vi "Create and Map Output Channel.vi"(8 "error in (no error)":errorcluster, 9 "Tag Name":string, 10 "engine":refnum<data-value>, 11 "E2E editor node in":refnum<data-value>) -> (0 "error out":errorcluster, 2 "engine out":refnum<data-value>, 3 "E2E editor node out":refnum<data-value>)   [LabVIEW 2015, in "E2E Tag Exchange editor node.lvclass"]
uses:
  E2E Tag Exchange editor node.lvclass
  <vilib>/NI/DCAF/Tag Editor Core/Configuration Editor/Classes/Engine Parent/Engine Parent Editor Node.lvclass
  <vilib>/NI/Tag Bus Module Framework/channel/channel classification.ctl
  E2E Tag Exchange editor node.lvclass/E2E Tag Exchange editor node.ctl
  <vilib>/NI/Tag Bus/tag/tag descriptor.lvclass/tag descriptor.ctl
  <vilib>/NI/Configuration Framework/serializable configuration/NISE_CEF_serializable configuration.lvclass/NISE_CEF_serializable configuration.ctl
  <vilib>/Utility/LVClass/Get LV Class Name.vi
  <vilib>/NI/Configuration Framework/error generator/NISE_error generator.vi
  <vilib>/NI/Module Execution Interface/Engine Configuration/engine configuration.lvclass
  module/configuration/E2E Tag Exchange configuration.lvclass
  <vilib>/NI/Tag Bus Module Framework/channel/TBM channel.lvclass
  <vilib>/NI/Tag Bus/tag/tag descriptor.lvclass
  <vilib>/NI/Configuration Framework/serializable configuration/NISE_CEF_serializable configuration.lvclass
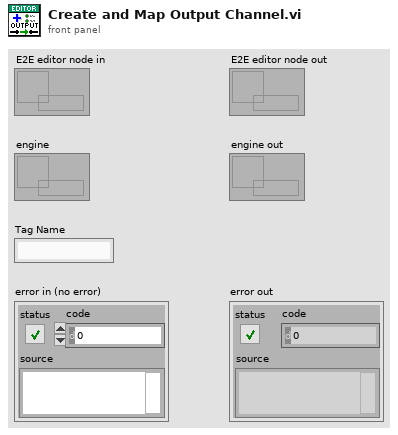
[diagram p1: front panel]
types:
  T1 = typedef "TBM channel.lvclass/channel classification.ctl" = enum16{"input data", "output data", "processing parameter", "processing result"}
  T2 = typedef "tag bus.lvlib/tag descriptor.lvclass/Data Type.ctl" = enum16{"Double", "Single", "I64", "I32", "I16", "I8", "U64", "U32", "U16", "U8", "Boolean", "String", "Array of Double", "Array of Single", "Array of I64", "Array of I32", "Array of I16", "Array of I8", "Array of U64", "Array of U32", "Array of U16", "Array of U8", "Array of Boolean", "Array of String"}
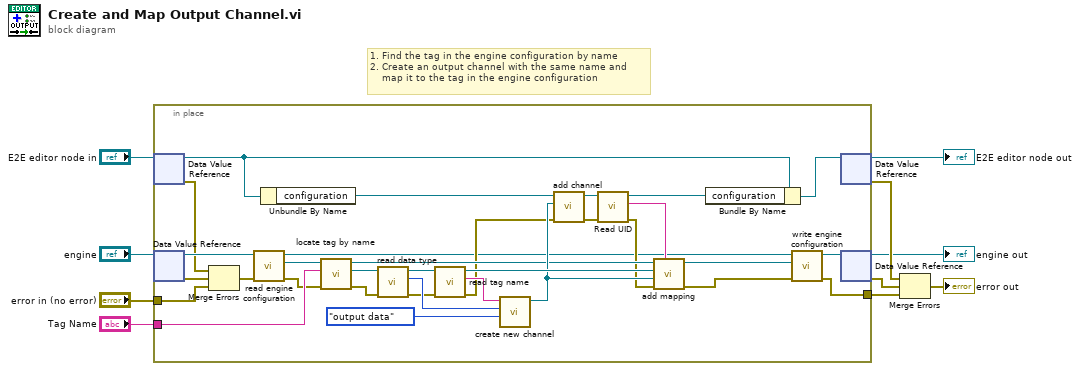
[diagram p0: block diagram]
diagram:
  # "1. Find the tag in the engine configuration by name\n2. Create an output channel with the same name and\n    map it to the tag in the engine configuration"
  n1 = in-place {
    in-place-border: "Tag Name" -> [w40]
    in-place-border: "error in (no error)" -> [w15]
    in-place-border: [w11] -> w6
    n2 = in-place-dvr #1("E2E editor node in") -> (w22:refnum<class "E2E Tag Exchange editor node.lvclass">, w12:errorcluster)
    n3 = in-place-dvr #2("engine") -> (w42:refnum<class "Engine Parent Editor Node.lvclass">, w14:errorcluster)
    n4 = Merge Errors(w12, w14, w15) -> (w13:errorcluster)
    n5 = call <vilib>:"read engine configuration.vi"("error in"=w13, "Engine Parent Editor Node in"=w42) -> ("error out"=w16:errorcluster, "engine configuration"=w41:refnum<class "engine configuration.lvclass">, "Engine Parent Editor Node out"=w19:refnum<class "Engine Parent Editor Node.lvclass">)  [unwired: 7 in]
    n6 = Unbundle By Name(w22) -> ("configuration"=w37:refnum<class "E2E Tag Exchange configuration.lvclass">)
    n7 = call <vilib>:"locate tag by name.vi"("error in"=w16, "tag name"=w40, "engine configuration in"=w41) -> ("error out"=w28:errorcluster, "tag descriptor"=w39:refnum<class "tag descriptor.lvclass">, "engine configuration out"=w31:refnum<class "engine configuration.lvclass">)  [unwired: 6 in]
    n8 = call <vilib>:"read data type.vi"("error in"=w28, "system tag in"=w39) -> ("error out"=w27:errorcluster, "data type"=w35:T2, "system tag out"=w38:refnum<class "tag descriptor.lvclass">)  [unwired: 7 in]
    n9 = call <vilib>:"read tag name.vi"("error in"=w27, "system tag in"=w38) -> ("error out"=w26:errorcluster, "name"=w36:string, "system tag out"=w33:refnum<class "tag descriptor.lvclass">)  [unwired: 7 in]
    n10 = call <vilib>:"create new channel.vi"("channel classification"=channel_classification."output data", "data type"=w35, "channel name"=w36) -> ("channel"=w32:refnum<class "TBM channel.lvclass">)  [unwired: 8 in]
    n11 = call "add channel.vi"("error in (no error)"=w26, "channel"=w32, "E2E configuration in"=w37) -> ("error out"=w25:errorcluster, "E2E configuration out"=w30:refnum<class "E2E Tag Exchange configuration.lvclass">)  [unwired: 7 in]
    n12 = call <vilib>:"Read UID.vi"("error in"=w25, "configuration in"=w30) -> ("error out"=w24:errorcluster, "instance id"=w29:string, "configuration out"=w23:refnum<class "E2E Tag Exchange configuration.lvclass">)  [unwired: 7 in]
    n13 = call-dynamic "add mapping.vi"("owner ID"=w29, "error in"=w24, "channel"=w32, "tag descriptor"=w33, "engine configuration"=w31) -> ("error out"=w17:errorcluster, "engine configuration out"=w18:refnum<class "engine configuration.lvclass">)  [unwired: 5 in]
    n14 = Bundle By Name(cluster=w22, "configuration"=w23) -> (w21:refnum<class "E2E Tag Exchange editor node.lvclass">)
    n15 = call <vilib>:"write engine configuration.vi"("error in"=w17, "engine configuration"=w18, "Engine Parent Editor Node in"=w19) -> ("error out"=w11:errorcluster, "Engine Parent Editor Node out"=w20:refnum<class "Engine Parent Editor Node.lvclass">)  [unwired: 7 in]
    n16 = in-place-dvr #1(w21) -> (→"E2E editor node out":refnum<data-value>, w4:errorcluster)
    n17 = in-place-dvr #2(w20) -> (→"engine out":refnum<data-value>, w5:errorcluster)
  }
  n18 = Merge Errors(w4, w5, w6) -> (→"error out":errorcluster)
